vi "to_json.vi"(8 "error in":errorcluster, 11 "gcs in":refnum<class "gcs.lvclass">) -> (0 "error out":errorcluster, 2 "json":string, 3 "gcs out":refnum<class "gcs.lvclass">, 4 "Not Default":bool)   [LabVIEW 2020, in "datasources.lvlib" / "gcs.lvclass"]
uses:
  gcs.lvclass
  C:/code/labview-client/lv_src/Nominal Client/datasources/source/source.lvclass
  source/source.lvclass/source.ctl
  d6cdba38-e6f4-4cfb-be00-b5423c713990.vi
  e4c6944f-4a67-449d-9f92-17c70d7df472.vi
  source/path.get.vi
  <vilib>/JDP Science/JSONtext/Variant to JSON Text.vi
  <vilib>/JDP Science/JSONtext/LVClass Serializer/JSONtext LVClass Serializer.lvclass
  gcs.lvclass/gcs.ctl
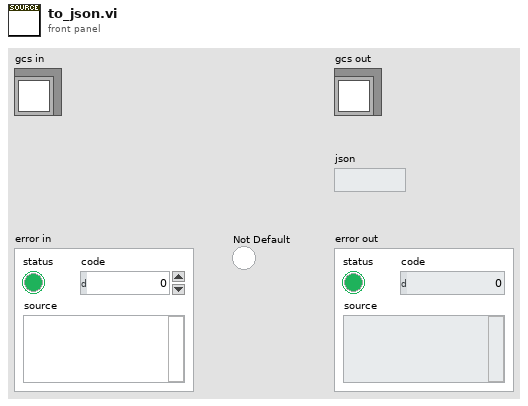
[diagram p1: front panel]
types:
  T1 = cluster{"type":string, "gcs":cluster{"path":string}}
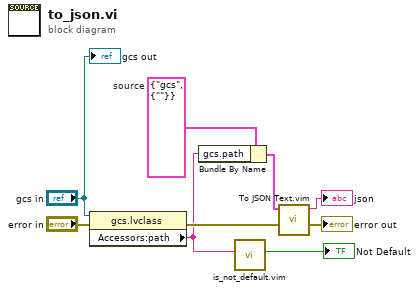
[diagram p0: block diagram]
diagram:
  w9 = T1 {"type"="gcs", "gcs"={"path"=""}}  # source
  n1 = property class="gcs.lvclass"(reference="gcs in", error in="error in") -> (error out=w7:errorcluster, "Accessors:path"=w1:string)  [unwired: 1 out]
  n2 = Bundle By Name(cluster=w9, "gcs.path"=w1) -> (w8:T1)
  n3 = call "is_not_default.vim"("data"=w1) -> ("Not Default"=→"Not Default":bool)  [unwired: 10 in]
  n4 = call "To JSON Text.vim"("error in (no error)"=w7, "Anything"=w8) -> ("error out"=→"error out":errorcluster, "<JSON>"=→"json":string)  [unwired: 8 in]
  "gcs out" <- "gcs in"
